vi "Read AppPath.vi"(8 "error in (no error)":errorcluster, 11 "UI_Actor in":refnum<class "UI_Actor.lvclass">) -> (0 "error out":errorcluster, 2 "AppPath":path, 3 "UI_Actor out":refnum<class "UI_Actor.lvclass">)   [LabVIEW 2020, in "UI_Actor.lvlib" / "UI_Actor.lvclass"]
doc: "In LabVIEW, c'est le chemin du dossier du launcher du root.\nIn EXE, c'est le chemin du dossier de l'executable."
uses:
  UI_Actor.lvclass
  UI_Actor.lvclass/UI_Actor.ctl
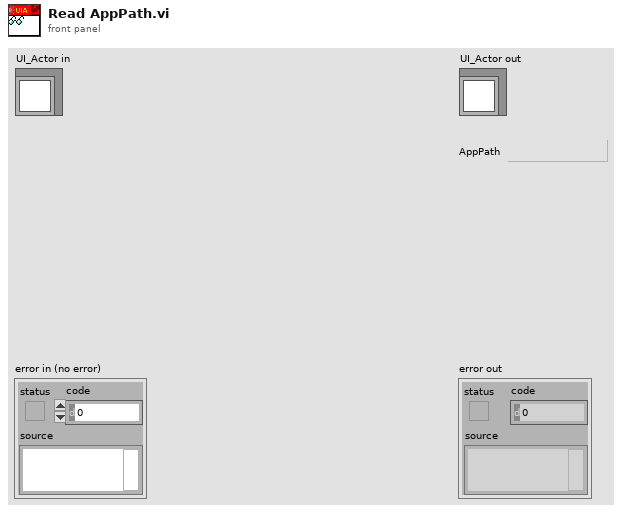
[diagram p1: front panel]
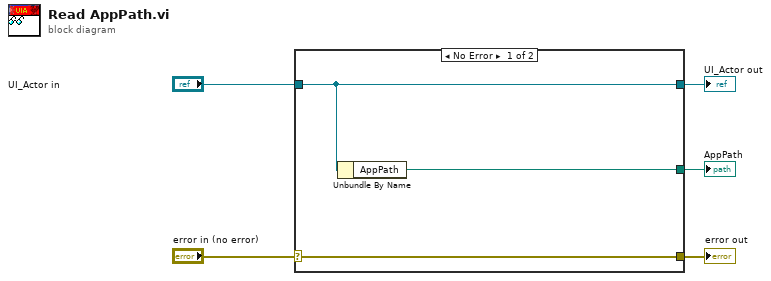
[diagram p0: block diagram]
diagram:
  n1 = case shown="No Error" "error in (no error)" {
    selector: "error in (no error)" -> [w8 w9]
    tunnel: [w8 w9] -> w4
    tunnel: [w7 w10] -> w2
    tunnel: "UI_Actor in" -> [w7 w10]
    tunnel: [w6 _] -> w1
    frame No Error {
      n2 = Unbundle By Name(w7) -> ("AppPath"=w6:path)
    }
    frame Error {
    }
  }
  "error out" <- w4
  "UI_Actor out" <- w2
  "AppPath" <- w1
